vi "Open Camera Quick Settings.vi"(8 "error in (no error)":errorcluster, 10 "SubPanel Ref":refnum<vi>, 11 "HIJ Vision Camera App in":refnum<class "HIJ Vision Camera App.lvclass">) -> (0 "error out":errorcluster, 3 "HIJ Vision Camera App out":refnum<class "HIJ Vision Camera App.lvclass">)   [LabVIEW 2014, in "HIJ Vision Camera App.lvlib" / "HIJ Vision Camera App.lvclass"]
uses:
  HIJ Vision Camera App.lvclass
  HIJ Vision Camera App.lvclass/HIJ Vision Camera App.ctl
  Camera Actors/IMAQdx Actor/IMAQdx Actor Messages/open camera quick settings Msg/open camera quick settings Msg.lvclass/open camera quick settings Msg.ctl
  <vilib>/ActorFramework/Message Enqueuer/Message Enqueuer.lvclass/Message Enqueuer.ctl
  <vilib>/ActorFramework/Message Enqueuer/Enqueue.vi
  <vilib>/ActorFramework/Message Priority Queue/Priority Enqueue.vi
  Camera Actors/IMAQdx Actor/IMAQdx Actor Messages/open camera quick settings Msg/open camera quick settings Msg.lvclass
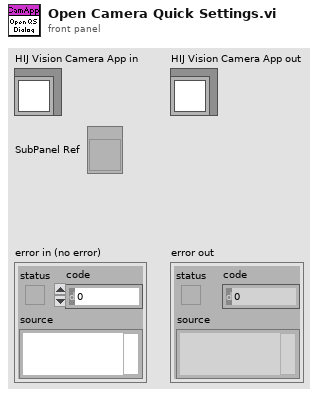
[diagram p1: front panel]
types:
  T1 = typedef "LVPositionTypeDef.ctl" = cluster{"Left":i32, "Top":i32}
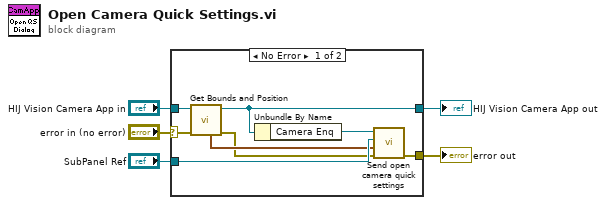
[diagram p0: block diagram]
diagram:
  n1 = case shown="No Error" "error in (no error)" {
    selector: "error in (no error)" -> [w7 w15]
    tunnel: [w11 w15] -> w4
    tunnel: [w6 w14] -> w2
    tunnel: "HIJ Vision Camera App in" -> [w8 w14]
    tunnel: "SubPanel Ref" -> [w12 _]
    frame No Error {
      n2 = call-dynamic "Get Bounds and Position.vi"("error in (no error)"=w7, "ViewableActor in"=w8) -> ("error out"=w9:errorcluster, "ViewableActor out"=w6:refnum<class "HIJ Vision Camera App.lvclass">, "Panel Position"=w10:T1)  [unwired: 5 in, 2 out]
      n3 = Unbundle By Name(w6) -> ("Camera Enq"=w13:refnum<class "Message Enqueuer.lvclass">)
      n4 = call "Send open camera quick settings.vi"("error in (no error)"=w9, "top left point"=w10, "SubPanel Ref"=w12, "Message Enqueuer"=w13) -> ("error out"=w11:errorcluster)  [unwired: 6 in, 1 out]
    }
    frame Error {
    }
  }
  "error out" <- w4
  "HIJ Vision Camera App out" <- w2
